vi "Send New Data.vi"(8 "error in (no error)":errorcluster, 10 "Channels":waveform(dbl)[](array[waveform]), 11 "MessageQ":refnum<class "MessageQ.lvclass">) -> (0 "error out":errorcluster)   [LabVIEW 2020, in "VolatusData.lvlib"]
uses:
  VolatusData.lvlib
  New Data.ctl
  Volatus/MessageQ/MessageQ.lvclass
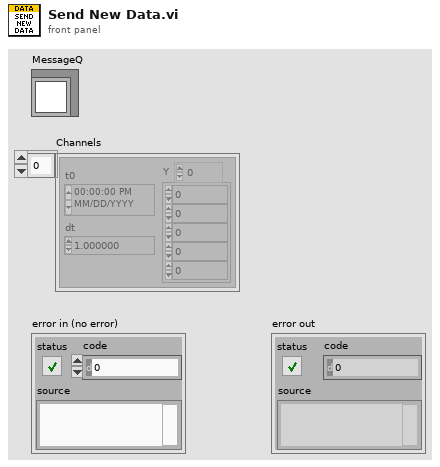
[diagram p1: front panel]
types:
  T1 = typedef "VolatusData.lvlib/New Data.ctl" = cluster{"Channels":waveform(dbl)[]}
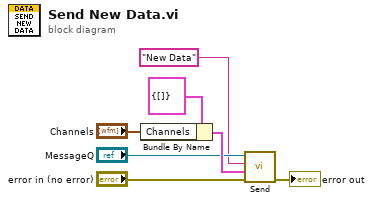
[diagram p0: block diagram]
diagram:
  n1 = Bundle By Name(cluster=T1 {"Channels"=[]} ("New Data"), "Channels"="Channels") -> (w4:T1)
  n2 = call "Send.vi"("error in (no error)"="error in (no error)", "Data"=w4, "ID"="New Data", "MessageQ in"="MessageQ") -> ("error out"=→"error out":errorcluster)  [unwired: 6 in, 1 out]
